vi "VI, Get Pane Origin.vi"(6 "error in":errorcluster, 8 "index (0)":i32, 9 "VI ref":refnum<vi>) -> (0 "error out":errorcluster, 3 "VI ref dup":refnum<vi>, 4 "y":i16, 5 "x":i16)   [LabVIEW 2010]
doc: "This function gets the origin (vertical and horizontal coordinates of the upper left corner of the pane) for one pane in a panel. The coordinates are relative to the coordinate system of the pane."
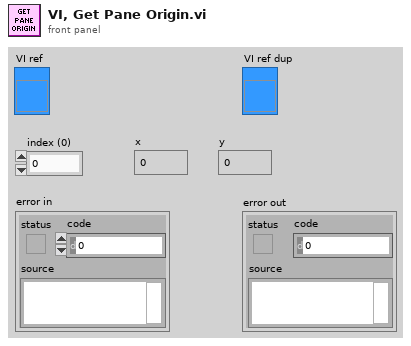
[diagram p1: front panel]
types:
  T1 = typedef "LVPointTypeDef.ctl" = cluster{"Horizontal":i16, "Vertical":i16}
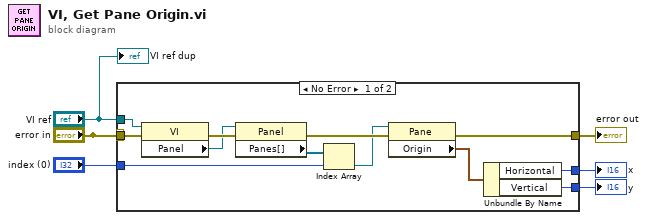
[diagram p0: block diagram]
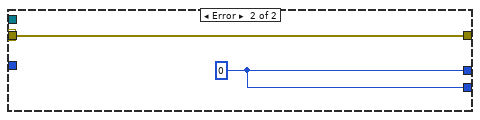
[diagram p2: hidden frame]
diagram:
  n1 = case shown="No Error" "error in" {
    selector: "error in" -> [_ w20]
    tunnel: [w10 w20] -> w6
    tunnel: "VI ref" -> [w17 _]
    tunnel: "error in" -> [w18 _]
    tunnel: "index (0)" -> [w12 _]
    tunnel: [w8 w19] -> w2
    tunnel: [w7 w19] -> w1
    frame No Error {
      n2 = property class="VI"(reference=w17, error in=w18) -> (error out=w16:errorcluster, "Panel"=w15:refnum<vi>)  [unwired: 1 out]
      n3 = property class="Panel"(reference=w15, error in=w16) -> (error out=w13:errorcluster, "Panes[]"=w14:refnum<vi>[])  [unwired: 1 out]
      n4 = Index Array(array=w14, index=w12) -> (element=w11:refnum<vi>)
      n5 = property class="Pane"(reference=w11, error in=w13) -> (error out=w10:errorcluster, "Origin"=w9:T1)  [unwired: 1 out]
      n6 = Unbundle By Name(w9) -> ("Horizontal"=w8:i16, "Vertical"=w7:i16)
    }
    frame Error {
      w19 = i16 0 ("Horizontal")
    }
  }
  "error out" <- w6
  "x" <- w2
  "y" <- w1
  "VI ref dup" <- "VI ref"
